vi "close.vi"(8 "error in (no error)":errorcluster caption="错误输入（无错误）", 11 "LXMCU_40G 输入":refnum<class "LXMCU_40G.lvclass"> caption="DNL_LabVIEW Object in") -> (0 "error out":errorcluster caption="错误输出", 3 "LXMCU_40G 输出":refnum<class "LXMCU_40G.lvclass"> caption="DNL_LabVIEW Object out")   [LabVIEW 2011, in "LXMCU_40G.lvclass"]
uses:
  LXMCU_40G.lvclass
  LXMCU_40G.lvclass/LXMCU_40G.ctl
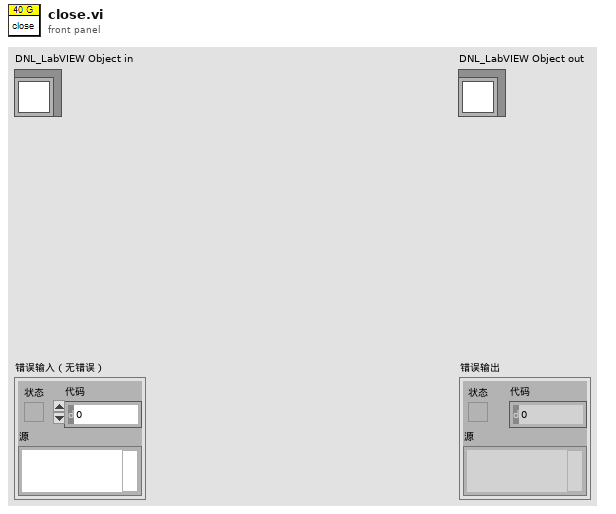
[diagram p1: front panel]
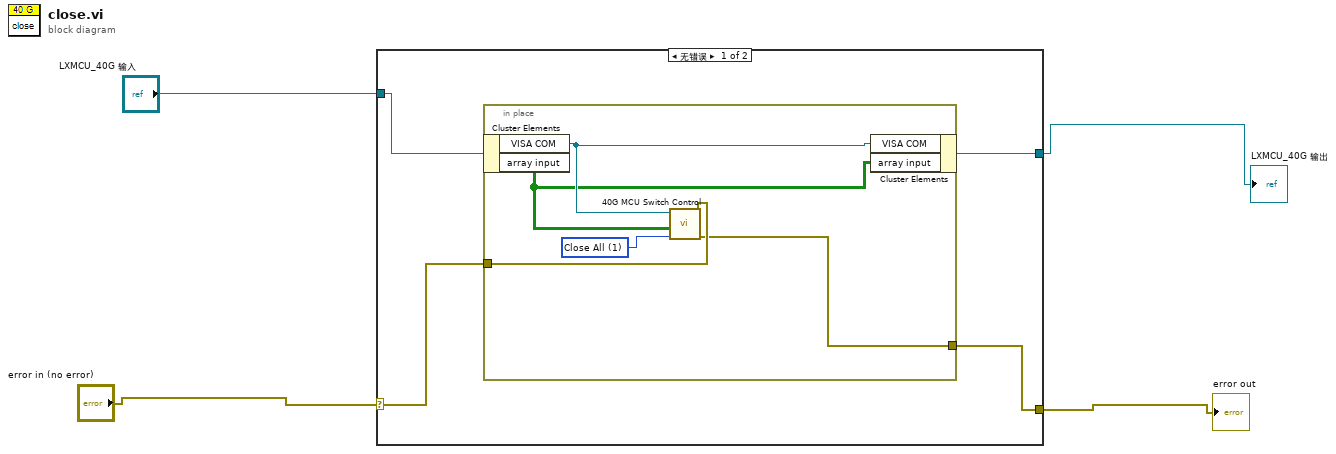
[diagram p0: block diagram]
diagram:
  n1 = case shown="无错误" "error in (no error)" {
    selector: "error in (no error)" -> [w7 w14]
    tunnel: "LXMCU_40G 输入" -> [w8 w15]
    tunnel: [w6 w14] -> w1
    tunnel: [w5 w15] -> w3
    frame No Error {
      n2 = in-place {
        in-place-border: w7 -> [w12]
        in-place-border: [w11] -> w6
        w13 = u16 1 items=["Testing", "Close All"] ("Function")
        n3 = in-place-cluster #1(w8) -> ("VISA COM"=w10:refnum<visa-resource-name>, "array input"=w9:bool[][])
        n4 = call "40G MCU Switch Control.vi"("Error in"=w12, "Function"=w13, "Array input:"=w9, "VISA"=w10) -> ("error out"=w11:errorcluster)  [unwired: 7 in]
        n5 = in-place-cluster #1("VISA COM"=w10, "array input"=w9) -> (w5:refnum<class "LXMCU_40G.lvclass">)
      }
    }
    frame Error {
    }
  }
  "error out" <- w1
  "LXMCU_40G 输出" <- w3
